vi "StableTemp.VI"(0 "GPIB Device":i16=15 min=1 max=32 step=1, 1 "Desired Temp":dbl=100.0 format="%.2f", 2 "Tolerance":dbl=1.0 min=0.01 max=500.0 format="%.2f", 3 "error in (no error)":errorcluster, 4 "AutoAdvancing":bool) -> (5 "Final Temp":sgl format="%.2f", 7 "error out":errorcluster)   [LabVIEW 2020]
doc: "This VI returns the reading from Sensor #1"
panel:
  in  "Time-out (S)":dbl=5.0 min=0.0 max=10000.0 format="%.2f"
  out "Temperature2":sgl(graph)
  out "Temperature1":sgl(graph)
  in  "Advancing?":bool
  out "GPIB Error code":i32
  # "Conductus LTC Get Temperature 1 VI"
  # "test"
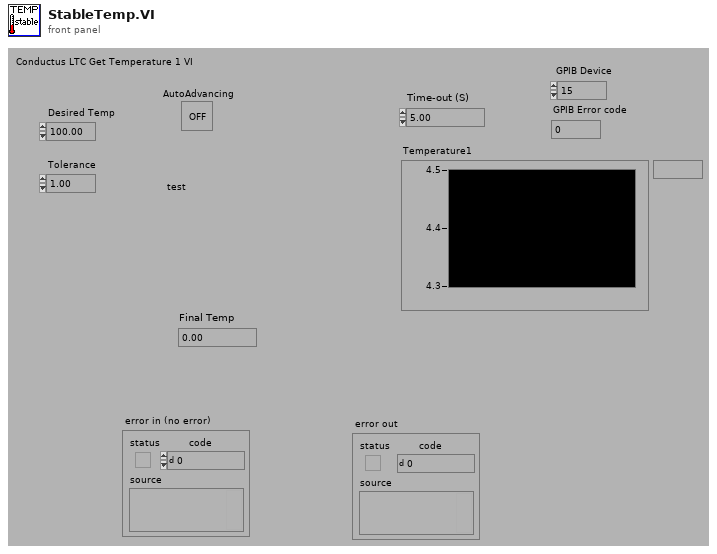
[diagram p1: front panel]
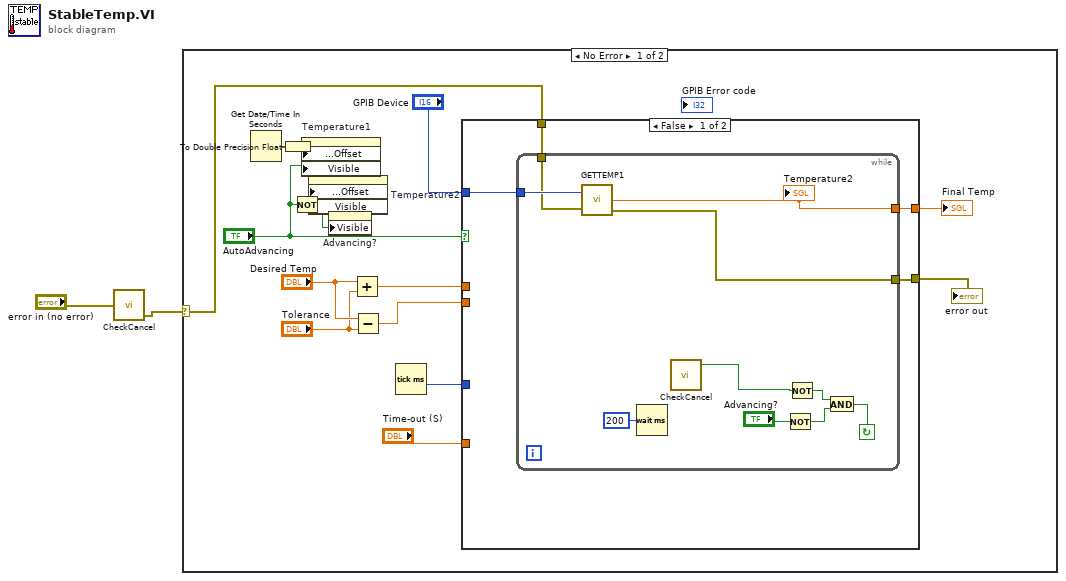
[diagram p0: block diagram]
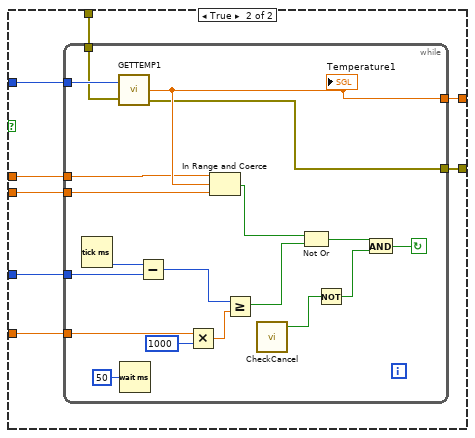
[diagram p2: hidden frame]
diagram:
  n1 = call "CheckCancel.vi"("error in (no error)"="error in (no error)") -> ("error out"=w2:errorcluster)  [unwired: 1 in, 1 out]
  n2 = case shown="No Error" w2 {
    selector: w2 -> [w3 _]
    frame No Error {
      n3 = Get Date/Time In Seconds() -> (seconds since 1Jan1904=w4:timestamp)
      n4 = To Double Precision Float(number=w4) -> (double precision float=w14:dbl)
      n5 = Not(x="AutoAdvancing") -> (.not. x?=w6:bool)
      n6 = property on="Temperature1" class="WFChart (strict)"("X Scale.Offset and Multiplier:Offset"=w14, "Visible"="AutoAdvancing") -> ()  [unwired: 2 in, 2 out]
      n7 = property on="Temperature2" class="WFChart (strict)"("X Scale.Offset and Multiplier:Offset"=w14, "Visible"=w6) -> ()  [unwired: 2 in, 2 out]
      n8 = property on="Advancing?" class="Bool"("Visible"=w6) -> ()  [unwired: 2 in, 2 out]
      n9 = Add(x="Desired Temp", y="Tolerance") -> (x+y=w8:dbl)
      n10 = Subtract(x="Desired Temp", y="Tolerance") -> (x-y=w7:dbl)
      n11 = Tick Count (ms)() -> (millisecond timer value=w12:u32)
      n12 = case shown="False" "AutoAdvancing" {
        tunnel: [w20 w38] -> w16
        tunnel: "GPIB Device" -> [w19 w37]
        tunnel: w12 -> [_ w36]
        tunnel: "Time-out (S)" -> [_ w35]
        tunnel: w8 -> [_ w34]
        tunnel: w7 -> [_ w33]
        tunnel: w3 -> [w18 w32]
        tunnel: [w17 w31] -> w5
        frame False {
          n13 = while {
            tunnel: [w25] -> w17
            tunnel: w18 -> [w26]
            tunnel: w19 -> [w27]
            tunnel: [w28] -> w20
            stop <- w24 continue-if-true
            n14 = call "GETTEMP1.VI"("GPIB Device"=w27, "error in (no error)"=w26) -> ("Sensor 1"=w28:sgl, "error out"=w25:errorcluster)  [unwired: 1 out]
            "Temperature2" <- w28
            n15 = Wait (ms)(milliseconds to wait=u32 200) -> ()  [unwired: 1 out]
            n16 = call "CheckCancel.vi"() -> ("Cancelled"=w21:bool)  [unwired: 2 in, 1 out]
            n17 = Not(x="Advancing?") -> (.not. x?=w22:bool)
            n18 = Not(x=w21) -> (.not. x?=w23:bool)
            n19 = And(x=w23, y=w22) -> (x .and. y?=w24:bool)
          }
        }
        frame True {
          n20 = while {
            tunnel: [w43] -> w31
            tunnel: w32 -> [w44]
            tunnel: w33 -> [w47]
            tunnel: w34 -> [w48]
            tunnel: w35 -> [w52]
            tunnel: w36 -> [w54]
            tunnel: w37 -> [w56]
            tunnel: [w49] -> w38
            stop <- w42 continue-if-true
            n21 = Tick Count (ms)() -> (millisecond timer value=w55:u32)
            n22 = call "GETTEMP1.VI"("GPIB Device"=w56, "error in (no error)"=w44) -> ("Sensor 1"=w49:sgl, "error out"=w43:errorcluster)  [unwired: 1 out]
            "Temperature1" <- w49
            n23 = Wait (ms)(milliseconds to wait=u32 50) -> ()  [unwired: 1 out]
            n24 = Subtract(x=w55, y=w54) -> (x-y=w51:u32)
            n25 = Multiply(x=w52, y=u32 1000) -> (x*y=w50:dbl)
            n26 = In Range and Coerce(upper limit=w48, x=w49, lower limit=w47) -> (In Range?=w46:bool)  [unwired: 1 out]
            n27 = Greater Or Equal?(x=w51, y=w50) -> (x >= y?=w45:bool)
            n28 = call "CheckCancel.vi"() -> ("Cancelled"=w39:bool)  [unwired: 2 in, 1 out]
            n29 = Not Or(1:w45, 2:w46) -> (0:w41:bool)
            n30 = Not(x=w39) -> (.not. x?=w40:bool)
            n31 = And(x=w41, y=w40) -> (x .and. y?=w42:bool)
          }
        }
      }
      "error out" <- w5
      "Final Temp" <- w16
    }
    frame Error {
    }
  }
